vi "XPath表达式.vi"(7 "添加的路径":path, 8 "error in (no error)":errorcluster, 11 "XPath expression":string caption="XPath表达式") -> (0 "error out":errorcluster, 3 "字符串与值[]":T1)   [LabVIEW 2016, in "斯坦道总氮.lvlib"]
uses:
  <vilib>/Utility/miscctls.llb/LVStringsAndValuesArrayTypeDef_U16.ctl
  <vilib>/xml/Load XML File.vi
  <vilib>/xml/Close Reference(Node).vi
  <vilib>/xml/NI_XML.lvlib
  <resource>/objmgr/DOMUserDefRef.rc
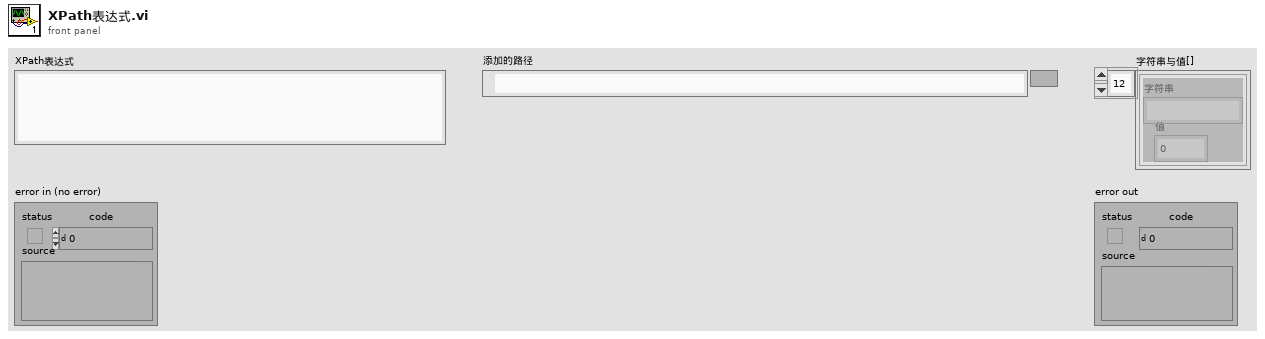
[diagram p1: front panel]
types:
  T1 = typedef "LVStringsAndValuesArrayTypeDef_U16.ctl" = cluster{"String":string, "Value":u16}[]
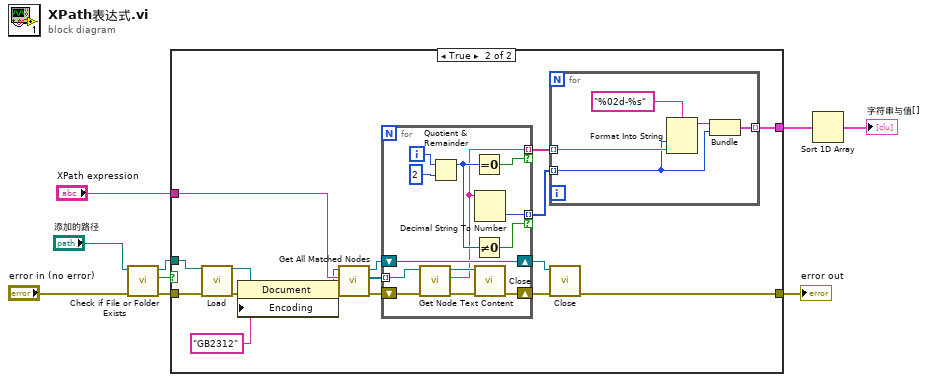
[diagram p0: block diagram]
diagram:
  n1 = call <vilib>:"Check if File or Folder Exists.vi"("error in (no error)"="error in (no error)", "path"="添加的路径") -> ("error out"=w5:errorcluster, "file or folder exists?"=w6:bool, "dup path"=w8:path)  [unwired: 7 in]
  n2 = case shown="True" w6 {
    tunnel: w8 -> [_ w27]
    tunnel: "XPath expression" -> [_ w21]
    tunnel: [_ w15] -> w2
    tunnel: w5 -> [w10 w12]
    tunnel: [w10 w11] -> w3
    frame False {
    }
    frame True {
      n3 = call-poly <vilib>:"Load.vi"("path to XML document"=w27, "error in (no error)"=w12) -> ("DOM document out"=w25:refnum<k20>, "error out"=w24:errorcluster)  [unwired: 11 in, 1 out]
      n4 = property on="属性节点" class="Document"(reference=w25, error in=w24, "Encoding"="GB2312" ("文档编码")) -> (reference out=w19:refnum<k20>, error out=w18:errorcluster)
      n5 = call <vilib>:"Get All Matched Nodes.vi"("error in (no error)"=w18, "XPath expression"=w21, "node in"=w19) -> ("error out"=w22:errorcluster, "node result array"=w23:refnum<k20>[], "node out"=w17:refnum<k20>)  [unwired: 6 in]
      n6 = for {
        tunnel: w23 -> [w41] mode=indexing
        shift-right: [w42] -> w20
        shift-left: w22 -> [w45]
        shift-right: [w40] -> w16
        shift-left: w17 -> [w40]
        tunnel: [w33] -> w14 mode=indexing if=w37
        tunnel: [w34] -> w13 mode=indexing if=w35
        i -> [w39]
        n7 = call <vilib>:"Get Node Text Content.vi"("error in (no error)"=w45, "node in"=w41) -> ("error out"=w43:errorcluster, "node text"=w33:string, "node out"=w44:refnum<k20>)  [unwired: 7 in]
        n8 = Quotient & Remainder(x=w39, y=2) -> (x-y*floor(x/y)=w36:i32)  [unwired: 1 out]
        n9 = Equal To 0?(x=w36) -> (x = 0?=w37:bool)
        n10 = Not Equal To 0?(x=w36) -> (x != 0?=w35:bool)
        n11 = Decimal String To Number(string=w33) -> (number=w34:i32)  [unwired: 2 in, 1 out]
        n12 = call-poly <vilib>:"Close.vi"("error in (no error)"=w43, "node"=w44) -> ("error out"=w42:errorcluster)  [unwired: 7 out]
      }
      n13 = for {
        tunnel: w14 -> [w30] mode=indexing
        tunnel: w13 -> [w28] mode=indexing
        tunnel: [w32] -> w15 mode=indexing
        n14 = Format Into String(format string="%02d-%s" ("格式字符串"), w28, w30) -> (resulting string=w29:string)  [unwired: 2 in, 1 out]
        n15 = Bundle(w29, w28) -> (w32:cluster{string, i32})  [unwired: 1 in]
      }
      n16 = call-poly <vilib>:"Close.vi"("error in (no error)"=w20, "node"=w16) -> ("error out"=w11:errorcluster)  [unwired: 7 out]
    }
  }
  "error out" <- w3
  n17 = Sort 1D Array(array=w2) -> (sorted array=→"字符串与值[]":cluster{string, i32}[])
